vi "Check Valid Direction.vi"(6 "Application out":refnum<class "Application.lvclass">, 7 "Pause/Resume Ref":refnum<vi>, 9 "Last Movement":T1=enum."Forward", 10 "ScanCode":i16, 11 "Current Direction":T1) -> (3 "New Direction":T1)   [LabVIEW 2021, in "Snake.lvclass"]
uses:
  Snake.lvclass
  GameEl_class/private/Enum Direction.ctl
  Application/Application.lvclass
  Application/Application.lvclass/Application.ctl
  Board Game_class/Board Game.lvclass/Board Game.ctl
  Application/Read Board Game.vi
  Board Game_class/Read Snake.vi
  Board Game_class/Board Game.lvclass
  GameEl_class/GameEl.lvclass
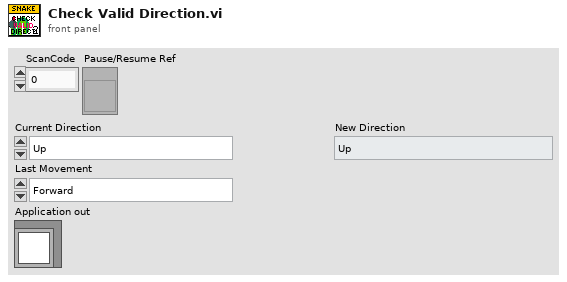
[diagram p1: front panel]
types:
  T1 = typedef "GameEl.lvclass/Enum Direction.ctl" = enum16{"Up", "Down", "Forward", "Backward"}
  T2 = typedef "Snake.lvclass/Snake Status.ctl" = cluster{"Boosters":cluster{"Shield":bool, "Star":bool}, "Weakeners":cluster{"Grapes":bool, "Bomb Crash":bool, "Death":bool}}
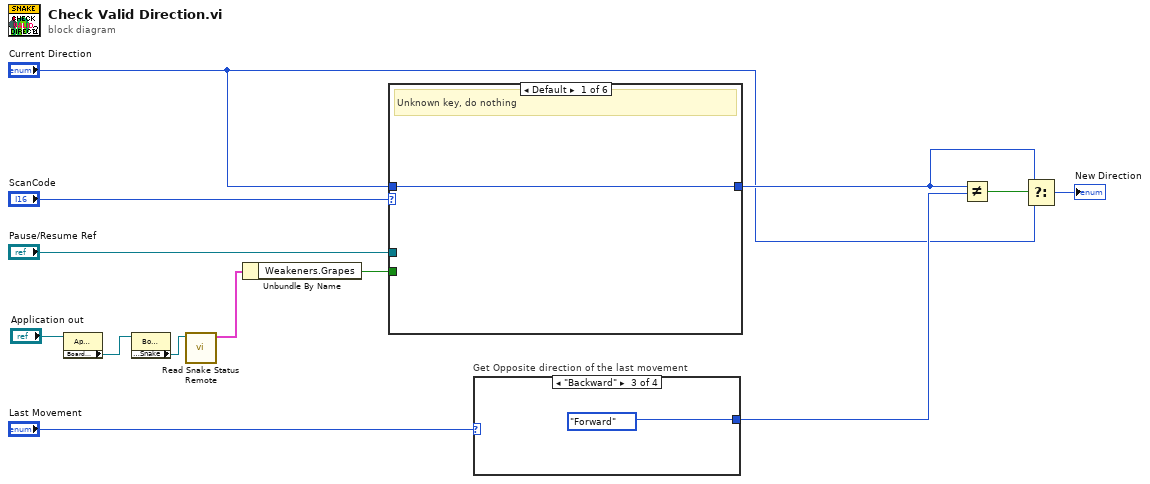
[diagram p0: block diagram]
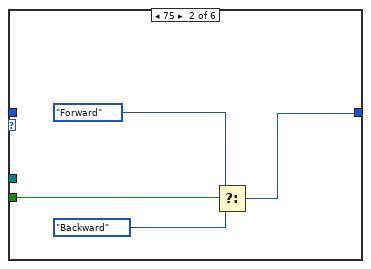
[diagram p2: hidden frame]
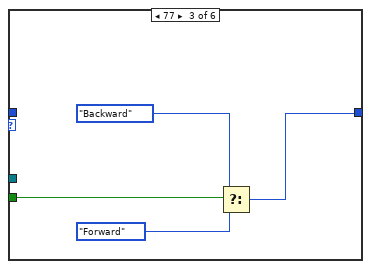
[diagram p3: hidden frame]
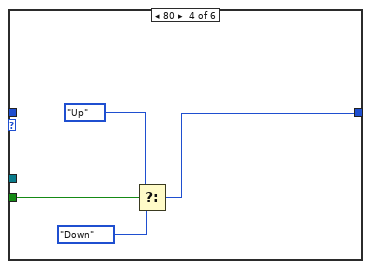
[diagram p4: hidden frame]
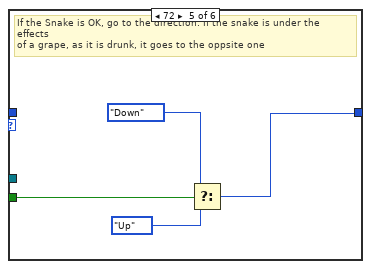
[diagram p5: hidden frame]
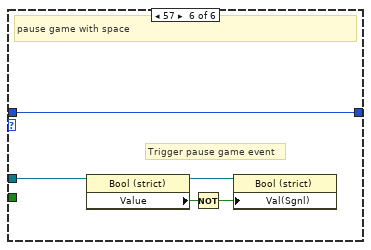
[diagram p6: hidden frame]
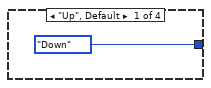
[diagram p7: hidden frame]
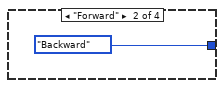
[diagram p8: hidden frame]
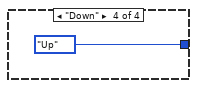
[diagram p9: hidden frame]
diagram:
  n1 = property class="Application.lvclass"(reference="Application out") -> ("Board Game"=w2:refnum<class "Board Game.lvclass">)  [unwired: 1 in, 2 out]
  n2 = property class="Board Game"(reference=w2) -> ("dataAccess:Snake"=w1:refnum<class "Snake.lvclass">)  [unwired: 1 in, 2 out]
  n3 = call "Read Snake Status Remote.vi"("Snake in"=w1) -> ("Snake Status"=w4:T2)  [unwired: 9 in, 1 out]
  n4 = Unbundle By Name(w4) -> ("Weakeners.Grapes"=w3:bool)
  n5 = case shown="Default" "ScanCode" {
    tunnel: [w14 w15 w19 w23 w27 w35] -> w8
    tunnel: "Current Direction" -> [w14 _ _ _ _ w35]
    tunnel: "Pause/Resume Ref" -> [_ _ _ _ _ w32]
    tunnel: w3 -> [_ w18 w22 w26 w30 _]
    frame Default {
      # "Unknown key, do nothing"
    }
    frame 75 {
      n6 = Select(t=Enum_Direction."Forward" ("Direction"), s=w18, f=Enum_Direction."Backward" ("Direction")) -> (s? t:f=w15:T1)
    }
    frame 77 {
      n7 = Select(t=Enum_Direction."Backward" ("Direction"), s=w22, f=Enum_Direction."Forward" ("Direction")) -> (s? t:f=w19:T1)
    }
    frame 80 {
      n8 = Select(t=Enum_Direction."Up" ("Direction"), s=w26, f=Enum_Direction."Down" ("Direction")) -> (s? t:f=w23:T1)
    }
    frame 72 {
      # "If the Snake is OK, go to the direction. If the snake is under the effects\nof a grape, as it is drunk, it goes to the oppsite one"
      n9 = Select(t=Enum_Direction."Down" ("Direction"), s=w30, f=Enum_Direction."Up" ("Direction")) -> (s? t:f=w27:T1)
    }
    frame 57 {
      # "Trigger pause game event"
      # "pause game with space"
      n10 = property on="Property Node" class="Bool (strict)"(reference=w32) -> (reference out=w31:refnum<vi>, "Value"=w34:bool)  [unwired: 1 in, 1 out]
      n11 = Not(x=w34) -> (.not. x?=w33:bool)
      n12 = property on="Property Node" class="Bool (strict)"(reference=w31, "Val(Sgnl)"=w33) -> ()  [unwired: 1 in, 2 out]
    }
  }
  n13 = case "Get Opposite direction of the last movement" shown="\"Backward\"" "Last Movement" {
    tunnel: [Enum_Direction."Down" ("Opposite Direction") Enum_Direction."Backward" ("Opposite Direction") Enum_Direction."Forward" ("Opposite Direction") Enum_Direction."Up" ("Opposite Direction")] -> w10
    frame "Up", Default {
    }
    frame "Forward" {
    }
    frame "Backward" {
    }
    frame "Down" {
    }
  }
  n14 = Not Equal?(x=w8, y=w10) -> (x != y?=w9:bool)
  n15 = Select(t=w8, s=w9, f="Current Direction") -> (s? t:f=→"New Direction":T1)
